vi "sabertooth packetized v3.vi"() -> ()   [LabVIEW 2018]
uses:
  package/controls/Sabertooth Baud Rate Select.ctl
panel:
  in  "stop":bool
  in  "Motor Speed 1":dbl(knob) scale=-1.0..1.0
  in  "Motor Speed 2":dbl(knob) scale=-1.0..1.0
  in  "Motor Speed 3":dbl(knob) scale=-1.0..1.0
  in  "Motor Speed 4":dbl(knob) scale=-1.0..1.0
  out "Loop Time":u32
  out "error out":errorcluster
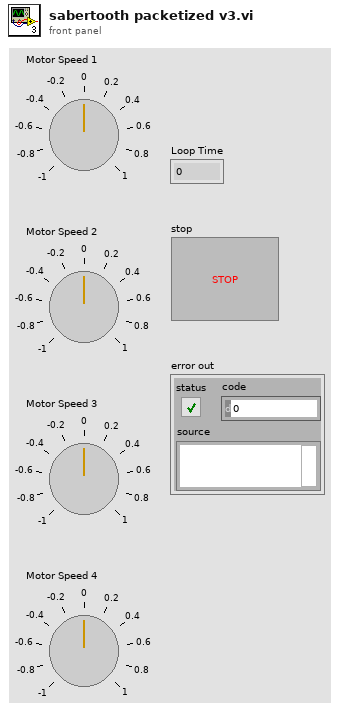
[diagram p1: front panel]
types:
  T1 = typedef "Sabertooth Baud Rate Select.ctl" = u32
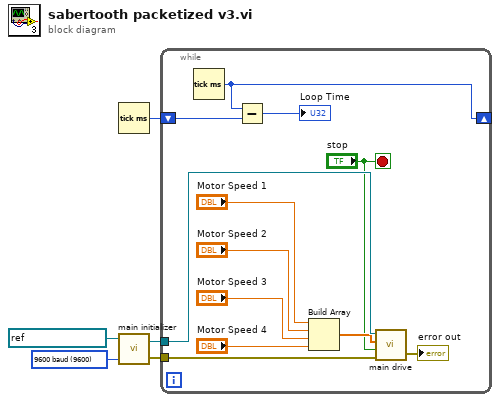
[diagram p0: block diagram]
diagram:
  w1 = T1 9600 items=["2400 baud"=2400, "9600 baud"=9600, "19200 baud"=19200, "38400 baud"=38400, "115200 baud"=115200] ("Current Baud Rate (115200)")
  n1 = Tick Count (ms)() -> (millisecond timer value=w5:u32)
  n2 = call "main initializer.vi"("Current Baud Rate (115200)"=w1, "VISA resource name in"=refnum<visa-resource-name> "ASRL1::INSTR") -> ("error out"=w3:errorcluster, "VISA resource name out"=w4:refnum<visa-resource-name>)  [unwired: 1 in]
  n3 = while {
    shift-right: [w11] -> _
    shift-left: w5 -> [w13]
    tunnel: w4 -> [w10]
    tunnel: w3 -> [w9]
    stop <- "stop" stop-if-true
    n4 = Tick Count (ms)() -> (millisecond timer value=w11:u32)
    n5 = Subtract(x=w11, y=w13) -> (x-y=→"Loop Time":u32)
    n6 = Build Array("Motor Speed 1", "Motor Speed 2", "Motor Speed 3", "Motor Speed 4") -> (w7:dbl[])
    n7 = call "main drive.vi"("error in (no error)"=w9, "Stop? (Speeds = 0?)"="stop", "Array of Motor Speeds"=w7, "VISA resource name"=w10) -> ("error out"=→"error out":errorcluster)  [unwired: 1 out]
  }
